vi "CheckDataVeto_FP_MON_CONN.vi"(0 "Connection ID TB":refnum<k5>, 1 "error in (no error)":errorcluster) -> (2 "concatenated string":string, 3 "PASS / FAIL":bool, 4 "error out":errorcluster)   [LabVIEW 2013]
panel:
  out "PROGRESS":i32(slide) scale=0.0..3.0
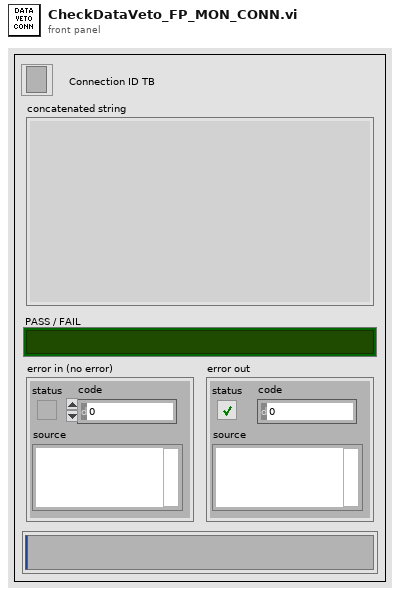
[diagram p1: front panel]
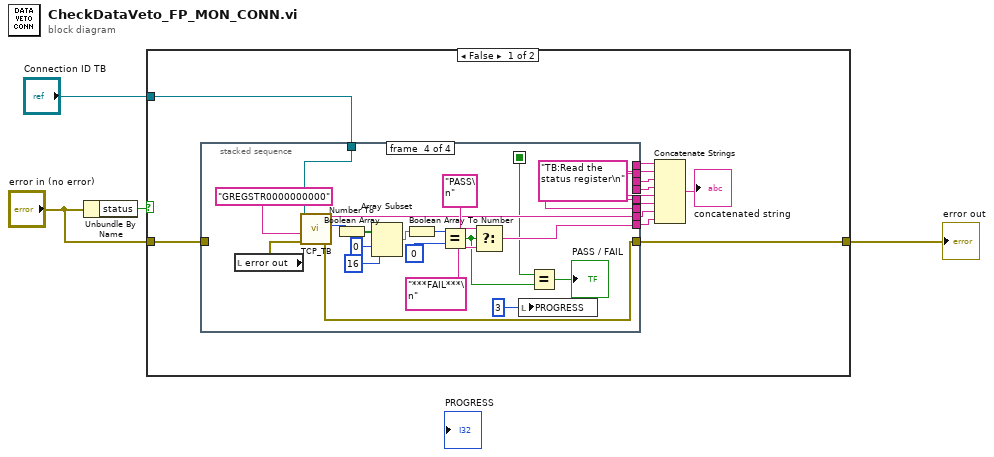
[diagram p0: block diagram]
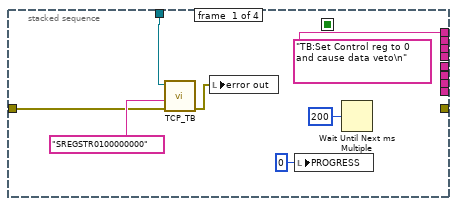
[diagram p2: hidden frame]
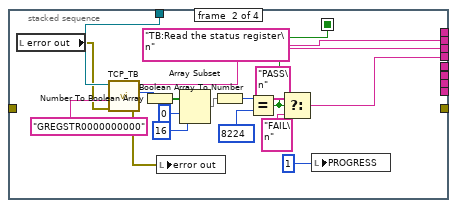
[diagram p3: hidden frame]
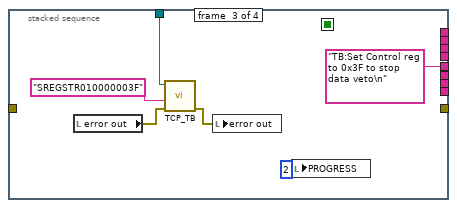
[diagram p4: hidden frame]
diagram:
  n1 = Unbundle By Name("error in (no error)") -> ("status"=w2:bool)
  n2 = case shown="False" w2 {
    tunnel: "Connection ID TB" -> [w7 _]
    tunnel: "error in (no error)" -> [w6 w68]
    tunnel: [w5 w68] -> w3
    frame False {
      n3 = stacked-sequence {
        seq-local: [_ w28 _ _] -> [_ _ _ w54]
        tunnel: ["TB:Set Control reg to 0 and cause data veto\n" ("COMMAND") _ _ _] -> w16
        tunnel: [_ "TB:Read the status register\n" ("COMMAND") _ _] -> w15
        tunnel: [_ w39 _ _] -> w14
        tunnel: [_ w29 _ _] -> w12
        tunnel: [_ _ "TB:Set Control reg to 0x3F to stop data veto\n" ("COMMAND") _] -> w11
        tunnel: [_ _ _ "TB:Read the status register\n" ("COMMAND")] -> w10
        tunnel: [_ _ _ w56] -> w8
        tunnel: [_ _ _ w55] -> w9
        tunnel: w7 -> [w19 w26 w44 w50]
        tunnel: w6 -> [w18 _ _ _]
        tunnel: [_ _ _ w49] -> w5
        frame #0 {
          n4 = call "TCP_TB.vi"("error in (no error)"=w18, "COMMAND"="SREGSTR0100000000", "Connection ID IN"=w19) -> ("error out"=w17:errorcluster)  [unwired: 3 in, 2 out]
          n5 = local write "error out"(w17) -> ()
          n6 = local write "PROGRESS"(0 ("PROGRESS")) -> ()
          n7 = Wait Until Next ms Multiple(millisecond multiple=u32 200) -> ()  [unwired: 1 out]
        }
        frame #1 {
          n8 = local read "error out"() -> (w25:errorcluster)
          n9 = call "TCP_TB.vi"("error in (no error)"=w25, "COMMAND"="GREGSTR0000000000", "Connection ID IN"=w26) -> ("error out"=w24:errorcluster, "Decimal Number"=w38:u32, "Their Response:"=w39:string)  [unwired: 3 in]
          n10 = Number To Boolean Array(number=w38) -> (Boolean array=w37:bool[])
          n11 = local write "error out"(w24) -> ()
          n12 = Array Subset(array=w37, index=0, length=16) -> (w34:bool[])
          n13 = Boolean Array To Number(Boolean array=w34) -> (number=w33:u32)
          n14 = Equal?(x=w33, y=u32 8224) -> (x = y?=w28:bool)
          n15 = Select(t="PASS\n" ("IP ADDRESS"), s=w28, f="FAIL\n" ("IP ADDRESS")) -> (s? t:f=w29:string)
          n16 = local write "PROGRESS"(1 ("PROGRESS")) -> ()
        }
        frame #2 {
          n17 = local read "error out"() -> (w43:errorcluster)
          n18 = call "TCP_TB.vi"("error in (no error)"=w43, "COMMAND"="SREGSTR010000003F", "Connection ID IN"=w44) -> ("error out"=w42:errorcluster)  [unwired: 3 in, 2 out]
          n19 = local write "error out"(w42) -> ()
          n20 = local write "PROGRESS"(2 ("PROGRESS")) -> ()
        }
        frame #3 {
          n21 = local read "error out"() -> (w48:errorcluster)
          n22 = call "TCP_TB.vi"("error in (no error)"=w48, "COMMAND"="GREGSTR0000000000", "Connection ID IN"=w50) -> ("error out"=w49:errorcluster, "Decimal Number"=w66:u32, "Their Response:"=w55:string)  [unwired: 3 in]
          n23 = Number To Boolean Array(number=w66) -> (Boolean array=w65:bool[])
          n24 = Array Subset(array=w65, index=0, length=16) -> (w62:bool[])
          n25 = Boolean Array To Number(Boolean array=w62) -> (number=w61:u32)
          n26 = Equal?(x=w61, y=u32 0) -> (x = y?=w53:bool)
          n27 = Select(t="PASS\n" ("IP ADDRESS"), s=w53, f="***FAIL***\n" ("IP ADDRESS")) -> (s? t:f=w56:string)
          n28 = local write "PROGRESS"(3 ("PROGRESS")) -> ()
          n29 = Equal?(x=w54, y=w53) -> (x = y?=→"PASS / FAIL":bool)
        }
      }
      n30 = Concatenate Strings(w16, w15, w14, w12, w11, w10, w9, w8) -> (→"concatenated string":string)
    }
    frame True {
    }
  }
  "error out" <- w3
